vi "writeMsg TEST.vi"() -> ()   [LabVIEW 2019]
uses:
  <vilib>/rvi/Emulation/niFpgaGetClockAttributes.vi
  <vilib>/rvi/Emulation/niFpgaSctlEmulationGetInTimedLoop.vi
  <vilib>/rvi/Emulation/niFpgaEmulationReportErrorSimple.vi
  <vilib>/rvi/Emulation/niFpgaCriticalErrorInLSC.vi
panel:
  in  "stop":bool
  in  "Frames to Write":u8
  in  "ID":u32 format="%x"
  in  "Data to Write":u8[](array[numeric])=[0, 0, 0, 0, 0, 0, 0, 0] format="%x"
  in  "ID Type":enum16{"Standard", "Extended"}(ring)
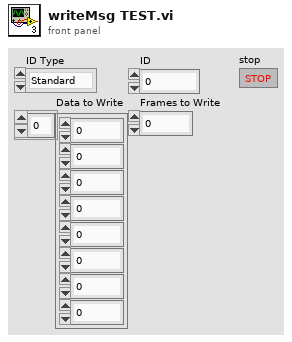
[diagram p1: front panel]
types:
  T1 = enum16{"100kBPS", "250kBPS", "500kBPS", "1000kBPS"}
  T2 = typedef "SPI Config.ctl" = cluster{"MXP Port":enum16{"A", "B"}, "Device":enum16{"CAN", "ENC", "IMU1", "IMU2"}, "CPOL":bool}
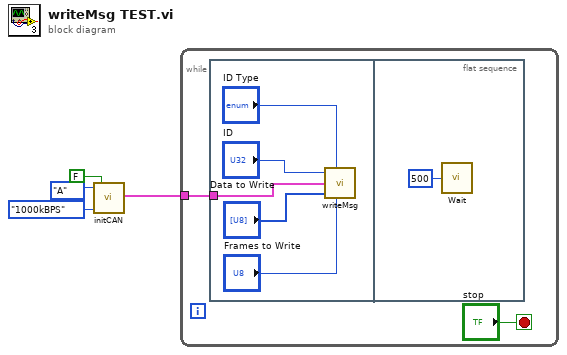
[diagram p0: block diagram]
diagram:
  n1 = call "initCAN.vi"("Baud Rate"=T1."1000kBPS", "CPOL"=FALSE, "MXP Port"=enum16{"A", "B"}."A") -> ("SPI Config Out"=w3:T2)
  n2 = while {
    tunnel: w3 -> [w6]
    stop <- "stop" stop-if-true
    n3 = flat-sequence {
      tunnel: w6 -> [w11]
      frame #0 {
        n4 = call "writeMsg.vi"("ID"="ID", "ID Type"="ID Type", "SPI Config In"=w11, "Data to Write"="Data to Write", "Frames to Write"="Frames to Write") -> ()  [unwired: 1 out]
      }
      frame #1 {
        n5 = call "Wait"("Count(mSec)"=u32 500) -> ()  [unwired: 1 out]
      }
    }
  }
